vi "_Axis_GetP.vi"(8 "Error In":errorcluster, 11 "轴序号":u16) -> (0 "Error Out":errorcluster, 3 "当前轴对应位置":i32)   [LabVIEW 2020, in "MT_API.lvlib"]
doc: "MT_API INT32 __stdcall MT_Get_Axis_Software_P_Now(WORD AObj,INT32* pValue);"
uses:
  MT_API.lvlib
  MT_API_64.dll
panel:
  out "函数返回值":i32
  # "获取对应轴的软件位置(脉冲个数)"
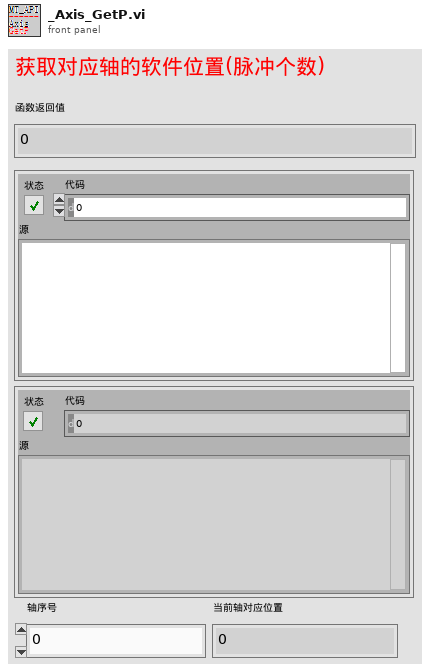
[diagram p1: front panel]
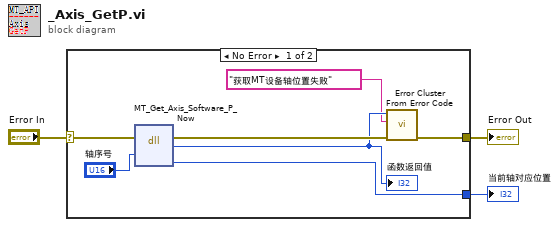
[diagram p0: block diagram]
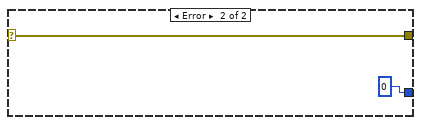
[diagram p2: hidden frame]
diagram:
  n1 = case shown="No Error" "Error In" {
    selector: "Error In" -> [w9 w12]
    tunnel: [w7 0] -> w2
    tunnel: [w4 w12] -> w1
    frame No Error {
      n2 = dll-call lib="D:/Project NJU/lib/MT/MT_API_64.*" fn="MT_Get_Axis_Software_P_Now"(error in=w9, "AObj"="轴序号") -> (error out=w8:errorcluster, "返回类型"=w6:i32, "pValue"=w7:i32)  [unwired: 4 in, 1 out]
      "函数返回值" <- w6
      n3 = call <vilib>:"Error Cluster From Error Code.vi"("error in (no error)"=w8, "error message (\"\")"="获取MT设备轴位置失败", "error code (0)"=w6) -> ("error out"=w4:errorcluster)  [unwired: 6 in]
    }
    frame Error {
    }
  }
  "Error Out" <- w1
  "当前轴对应位置" <- w2
